vi "Lighting Off.vi"(8 "error in (no error)":errorcluster, 11 "Root Object In":refnum<vi>) -> (0 "error out":errorcluster, 3 "Root Object Out":refnum<vi>)   [LabVIEW 2020, in "3D Plot.lvclass"]
uses:
  <vilib>/Math Plots/3D Math Plots/3D Plot/3D Plot/3D Plot.lvclass
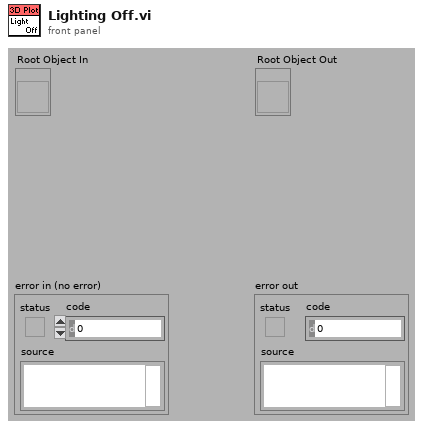
[diagram p1: front panel]
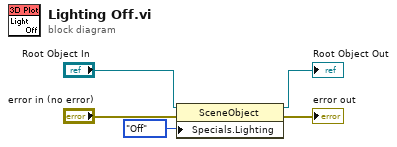
[diagram p0: block diagram]
diagram:
  n1 = property class="SceneObject"(reference="Root Object In", error in="error in (no error)", "Specials.Lighting"=enum16{"Inherit Value", "Off", "On"}."Off" ("Specials:Lighting")) -> (reference out=→"Root Object Out":refnum<vi>, error out=→"error out":errorcluster)
